vi "Case_Calc.vi"() -> ()   [LabVIEW 2018]
panel:
  in  "열거형":enum16{"더하기", "빼기", "곱하기", "나누기"}(ring)
  out "숫자형 3":dbl format="%#_13g"
  in  "숫자형 2":i32
  in  "숫자형":i32
  in  "콤보 박스":string(combo)="더하기"
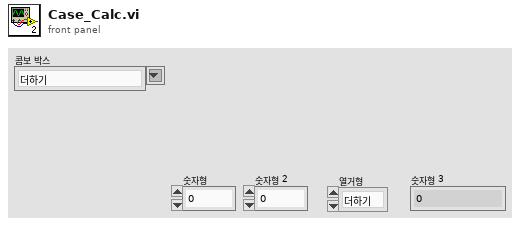
[diagram p1: front panel]
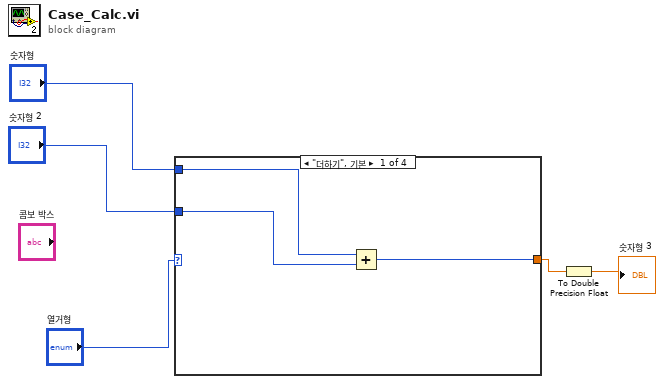
[diagram p0: block diagram]
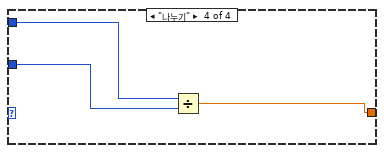
[diagram p4: hidden frame]
diagram:
  n1 = case shown="\"더하기\", 기본" "열거형" {
    tunnel: "숫자형" -> [w8 w9 _ w13]
    tunnel: "숫자형 2" -> [w7 _ w10 w12]
    tunnel: [w6 w9 w10 w11] -> w2
    frame "더하기", Default {
      n2 = Add(x=w8, y=w7) -> (x+y=w6:i32)
    }
    frame "빼기" {
    }
    frame "곱하기" {
    }
    frame "나누기" {
      n3 = Divide(x=w13, y=w12) -> (x/y=w11:dbl)
    }
  }
  n4 = To Double Precision Float(number=w2) -> (double precision float=→"숫자형 3":dbl)
